vi "MW_motion.vi"() -> ()   [LabVIEW 2018]
panel:
  in  "Tab Control":enum32{"Config", "UI"}(tab)=enum."UI"
  in  "com":refnum<visa-resource-name>="COM6"
  in  "write":bool=TRUE
  in  "baud":u32=115200
  in  "clr":bool
  in  "cmdsel":bool
  in  "strcmd":string="sp=1"
  in  "wait":u32=15
  out "concatenated string":string
  out "iter":i32=2973
  out "read buffer":string="pc1=25\r\n"
  out "pos Chart":cluster{i32, "Slide":i16}(graph)={25, "Slide"=25}
  in  "stop":bool
  in  "Slide":i16(slide)=25 scale=-2000.0..2000.0
  # "NTREX MW DCS01 demo"
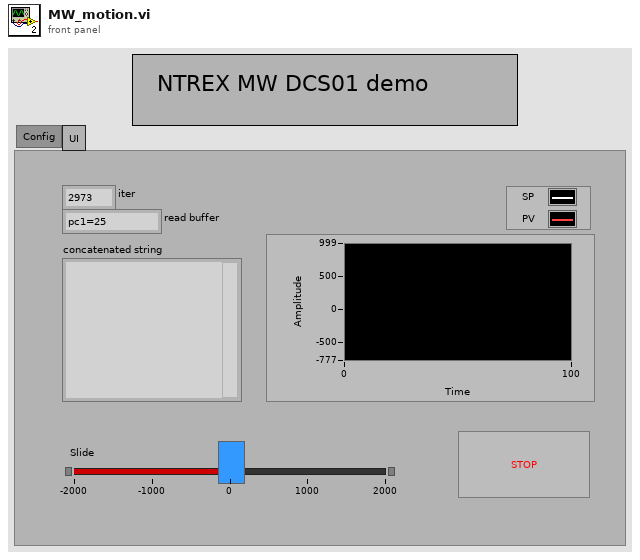
[diagram p1: front panel]
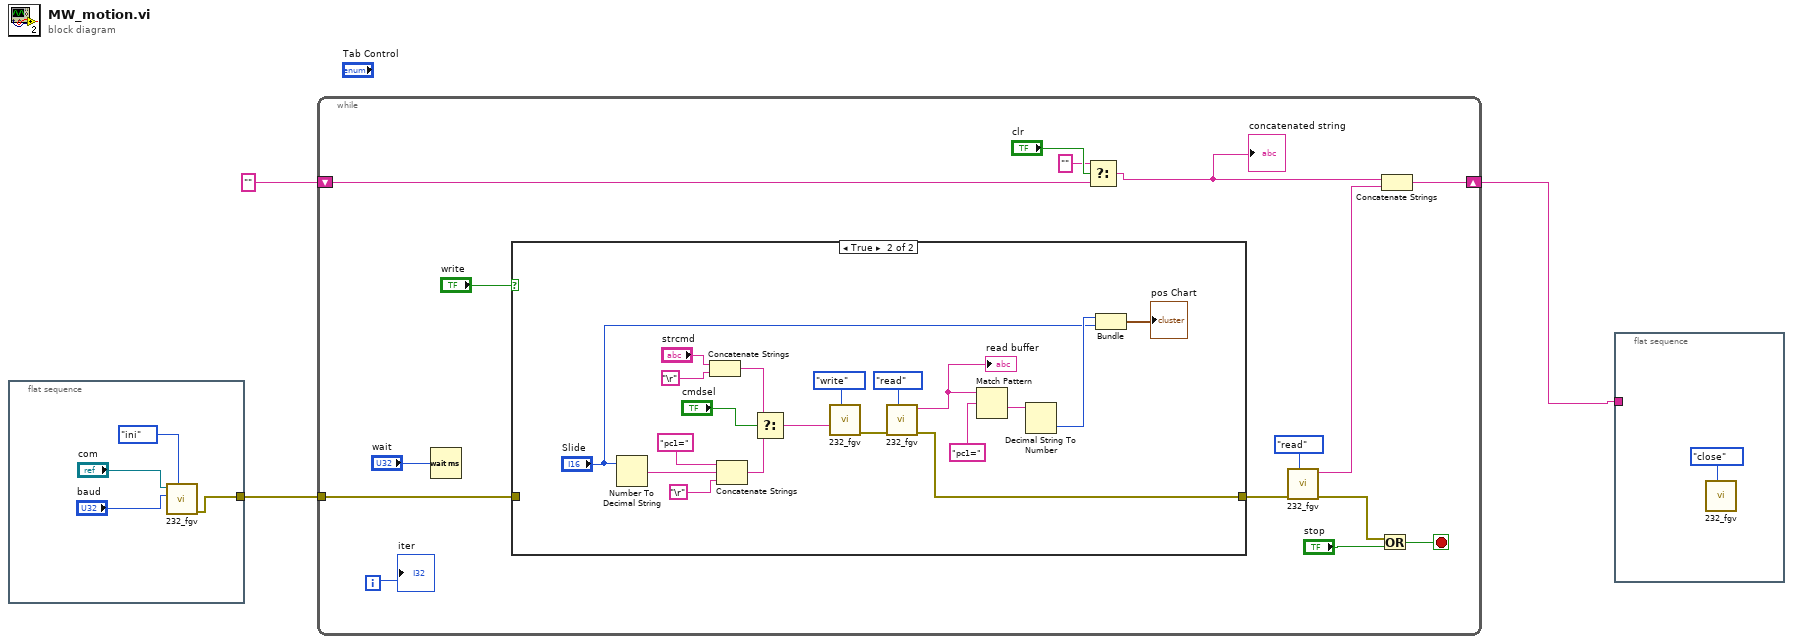
[diagram p0: block diagram]
diagram:
  n1 = flat-sequence {
    tunnel: [w5] -> w2
    frame #0 {
      n2 = call "232_fgv.vi"("cmd"=enum16{"close", "ini", "read", "write"}."ini", "baud rate (9600)"="baud", "VISA resource name"="com") -> ("error out"=w5:errorcluster)  [unwired: 7 in, 1 out]
    }
  }
  n3 = while {
    shift-right: [w21] -> w1
    shift-left: "" -> [w16]
    tunnel: w2 -> [w11]
    i -> [w18]
    stop <- w9 stop-if-true
    n4 = Wait (ms)(milliseconds to wait="wait") -> ()  [unwired: 1 out]
    n5 = case shown="True" "write" {
      tunnel: [w23 w24] -> w13
      tunnel: w11 -> [w23 _]
      frame False {
      }
      frame True {
        n6 = Number To Decimal String(number="Slide") -> (decimal integer string=w39:string)  [unwired: 1 in]
        n7 = Concatenate Strings("strcmd", "\r") -> (w30:string)
        n8 = Concatenate Strings("pc1=" ("strcmd"), w39, "\r") -> (w40:string)
        n9 = Select(t=w30, s="cmdsel", f=w40) -> (s? t:f=w28:string)
        n10 = call "232_fgv.vi"("cmd"=enum16{"close", "ini", "read", "write"}."write", "write buffer"=w28) -> ("error out"=w26:errorcluster)  [unwired: 8 in, 1 out]
        n11 = call "232_fgv.vi"("cmd"=enum16{"close", "ini", "read", "write"}."read", "error in"=w26) -> ("error out"=w24:errorcluster, "read buffer"=w25:string)  [unwired: 8 in]
        "read buffer" <- w25
        n12 = Match Pattern(string=w25, regular expression="pc1=") -> (after substring=w37:string)  [unwired: 1 in, 3 out]
        n13 = Decimal String To Number(string=w37) -> (number=w36:i32)  [unwired: 2 in, 1 out]
        n14 = Bundle(w36, "Slide"="Slide") -> (→"pos Chart":cluster{i32, "Slide":i16})  [unwired: 1 in]
      }
    }
    n15 = Select(t="", s="clr", f=w16) -> (s? t:f=w8:string)
    "concatenated string" <- w8
    n16 = call "232_fgv.vi"("cmd"=enum16{"close", "ini", "read", "write"}."read", "error in"=w13) -> ("error out"=w10:errorcluster, "read buffer"=w12:string)  [unwired: 8 in]
    n17 = Or(x=w10, y="stop") -> (x .or. y?=w9:bool)
    n18 = Concatenate Strings(w8, w12) -> (w21:string)
    "iter" <- w18
  }
  n19 = flat-sequence {
    tunnel: w1 -> [_]
    frame #0 {
      n20 = call "232_fgv.vi"("cmd"=enum16{"close", "ini", "read", "write"}."close") -> ()  [unwired: 9 in, 2 out]
    }
  }
